vi "TSM Relay Configuration Control.vi"(0 "Relay Configuration In":T1 {"Relay Action Configuration"."Relay Action" items=["Open Relay"=20, "Close Relay"=21]}, 2 "Settling Time (s)":dbl, 11 "error in (no error)":errorcluster) -> (15 "error out":errorcluster)   [LabVIEW 2020]
doc: "Performs the actions specified by the relay configuration."
uses:
  Pin Map/TSM Relay Configuration.ctl
  <vilib>/NI_TestStand_SemiconductorModule/NI_TestStand_Semiconductor_Module.lvlibp/PinMap/General/SemiconductorModuleContext.ctl
  Pin Map/TSM Relay to Action Map.ctl
  <vilib>/NI_TestStand_SemiconductorModule/NI_TestStand_Semiconductor_Module.lvlibp/1abvi3w/instr.lib/niSwitch/niswitch.llb/niSwitch Relay Action.ctl
  <vilib>/NI_TestStand_SemiconductorModule/NI_TestStand_Semiconductor_Module.lvlibp/PinMap/Relay Driver/ControlRelaysMultipleActions.vi
  <vilib>/NI_TestStand_SemiconductorModule/NI_TestStand_Semiconductor_Module.lvlibp
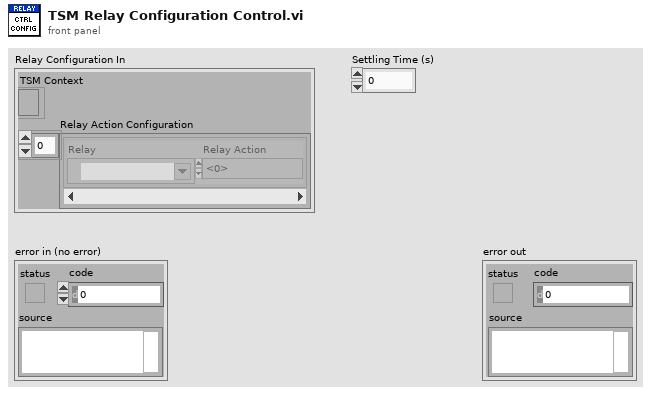
[diagram p1: front panel]
types:
  T1 = typedef "TSM Relay Configuration.ctl" = cluster{"TSM Context":T2, "Relay Action Configuration":T3[]}
  T2 = typedef "NI_TestStand_Semiconductor_Module.lvlibp/SemiconductorModuleContext.ctl" = refnum<k7>
  T3 = typedef "TSM Relay to Action Map.ctl" = cluster{"Relay":tag, "Relay Action":T4}
  T4 = typedef "NI_TestStand_Semiconductor_Module.lvlibp/niSwitch Relay Action.ctl" = i32
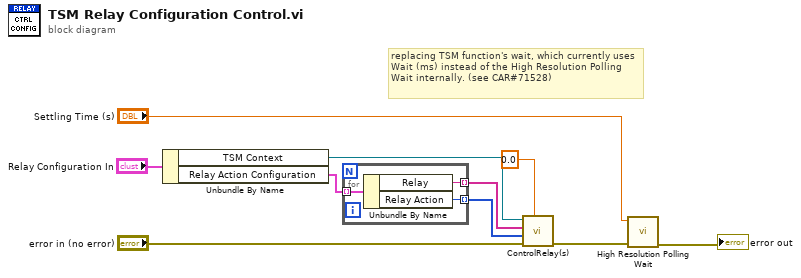
[diagram p0: block diagram]
diagram:
  # "replacing TSM function's wait, which currently uses Wait (ms) instead of the High Resolution Polling Wait internally. (see CAR#71528)"
  n1 = Unbundle By Name("Relay Configuration In") -> ("TSM Context"=w9:T2, "Relay Action Configuration"=w3:T3[])
  n2 = for {
    tunnel: [w13] -> w2 mode=indexing
    tunnel: [w12] -> w1 mode=indexing
    tunnel: w3 -> [w11] mode=indexing
    n3 = Unbundle By Name(w11) -> ("Relay"=w13:tag, "Relay Action"=w12:T4)
  }
  n4 = call-poly <vilib>:"ControlRelay(s).vi"("Wait (s)"=0.0, "error in (no error)"="error in (no error)", "Relay Actions"=w1, "Relays"=w2, "Semiconductor Module Context"=w9) -> ("error out"=w6:errorcluster)  [unwired: 5 in, 1 out]
  n5 = call <vilib>:"High Resolution Polling Wait.vi"("error in (no error)"=w6, "seconds to wait"="Settling Time (s)") -> ("error out"=→"error out":errorcluster)  [unwired: 9 in]
